vi "Scale Filter before Targeting to FXP.vi"() -> ()   [LabVIEW 2023]
doc: "Demonstrates how to use the DFD Scale Filter VI to scale the coefficients of a filter that has an IIR Cascaded Second-Order Sections Form structure. By scaling the filter coefficients, you can achieve an optimal fixed-point filter design.\n\nComplete the following steps to use this VI.\n1) Specify an IIR Cascaded Second-Order Sections Form structure in the <B>Target Structure</B> input.\n2) Verify that the <B>Scale Filter?</B> value is False.\n3) Run the VI.\n4) Observe the magnitude response, mean squared error (MSE) value, and coefficients report.\n5) Set the <B>Scale Filter?</B> value to True.\n6) Run this VI again. \n7) Observe the MSE value and coefficients report to learn the effect of scaling the filter coefficients before quantizing and modeling a fixed-point filter."
uses:
  <vilib>/addons/Digital Filter Design/_Objects.llb/DFD Quantization Sources.ctl
  <vilib>/addons/Digital Filter Design/_Objects.llb/DFD Coef Norm Type.ctl
  <vilib>/addons/Digital Filter Design/FXPModel.llb/DFD FXP Quantize Coef (Easy).vi
  <vilib>/addons/Digital Filter Design/Analysis.llb/DFD Plot Freq Response (Linear-Spaced).vi
  <vilib>/addons/Digital Filter Design/FXPModel.llb/DFD FXP Get Quantizer (One).vi
  <vilib>/addons/Digital Filter Design/Process.llb/DFD Filtering (Array).vi
  <vilib>/Utility/VariantDataType/GetNumericFxpInfo.vi
  <vilib>/addons/Digital Filter Design/FXPSim.llb/dfd_Check Input FXP Settings.vi
  <vilib>/addons/Digital Filter Design/FXPSim.llb/dfd_Check SRate Simulation Integer Input.vi
  <vilib>/addons/Digital Filter Design/FXPSim.llb/dfd_FXP Simu.vi
  <vilib>/addons/Digital Filter Design/_Objects.llb/DFD FXP Statistics Data.ctl
  <vilib>/addons/Digital Filter Design/FXPSim.llb/SimXnode/DFD FXP Simulation.xnode
  <vilib>/addons/Digital Filter Design/_Objects.llb/DFD Filter Obj.ctl
  <vilib>/addons/Digital Filter Design/_Objects.llb/DFD Filter Coef.ctl
  <vilib>/addons/Digital Filter Design/_Objects.llb/DFD Filter Structure Type Selector.ctl
  <vilib>/addons/Digital Filter Design/_Objects.llb/dfd_Internal Quantization Settings.ctl
  <vilib>/addons/Digital Filter Design/_Objects.llb/dfd_Internal Quantization Srcs.ctl
  <vilib>/addons/Digital Filter Design/NI_DigFilterLicensed.lvlib
  <vilib>/Analysis/NI_AALPro.lvlib
  <vilib>/Analysis/NI_AALBase.lvlib
  <vilib>/addons/Digital Filter Design/NI_DigFilter_FXP.lvlib
  <vilib>/Utility/VariantDataType/VariantType.lvlib
panel:
  out "MSE":dbl format="%.6g"
  out "Coefficients Report":string
  out "Magnitude Response":cluster{"f0":dbl, "df":dbl, "values":dbl[]}[](graph)
  in  "Scale Filter?":bool
  out "Error Message":string
  in  "Target Structure":u16(ring)=12 items=["FIR Direct Form"=1, "FIR Direct Form Transposed"=2, "FIR Symmetric"=3, "FIR Antisymmetric"=4, "IIR Direct Form I"=5, "IIR Direct Form I Transposed"=6, "IIR Direct Form II"=7, "IIR Direct Form II Transposed"=8, "IIR Cascaded Second-Order Sections Form I"=9, "IIR Cascaded Second-Order Sections Form I Transposed"=10, "IIR Cascaded Second-Order Sections Form II"=11, "IIR Cascaded Second-Order Sections Form II Transposed"=12, "Lattice Allpass (basic sections)"=13, "Lattice Allpass (one multiplier sections)"=14, "Lattice Allpass (normalized sections)"=15, "Lattice AR (basic sections)"=16, "Lattice AR (one multiplier sections)"=17, "Lattice AR (normalized sections)"=18, "Lattice MA (minimum phase)"=19, "Lattice MA (maximum phase)"=20, "Lattice ARMA (basic sections)"=21, "Lattice ARMA (one multiplier sections)"=22, "Lattice ARMA (normalized sections)"=23]
  out "Filtering Results":dbl[][](graph)
  # "Select Help>>Show Context Help and move the cursor over the VI icon for more information."
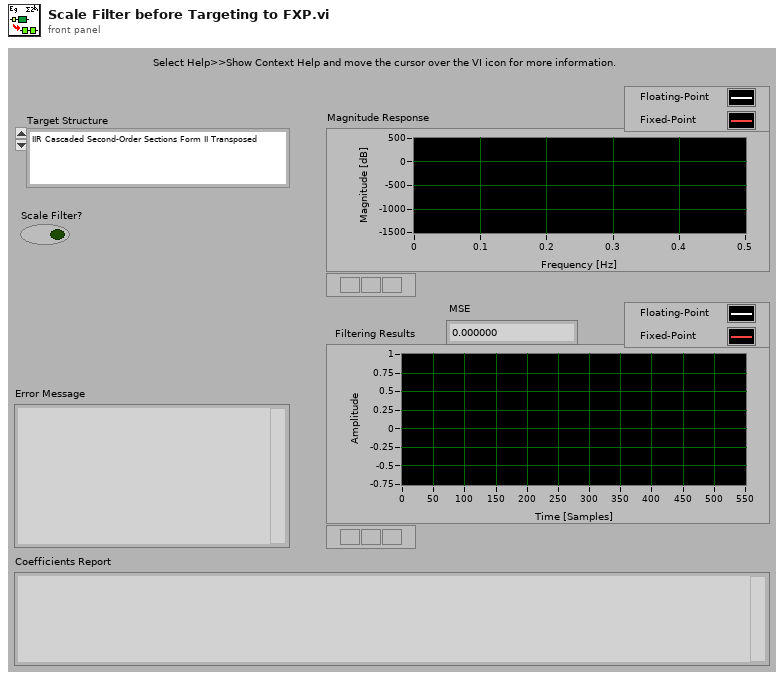
[diagram p1: front panel]
types:
  T1 = typedef "NI_DigFilterLicensed.lvlib/DFD Quantization Sources.ctl" = u16
  T2 = typedef "NI_DigFilterLicensed.lvlib/DFD Filter Obj.ctl" = cluster{"mSRate_Fs":dbl, "mSRate_Version":string, "mSRate_Comments":string, "mSRate_OrgCoef":T3, "mSRate_CurCoef":T3, "mSRate_Quantized?":bool, "mSRate_QCoef":T3, "mSRate_QSettings":T5[], "mSRate_Order":i32, "mSRate_Scaling":cluster{"mSRate_ScaleByPowerOf2?":bool, "mSRate_ScaleType":T7}}
  T3 = typedef "NI_DigFilterLicensed.lvlib/DFD Filter Coef.ctl" = cluster{"type":T4, "gain":dbl, "coef a (k)":dbl[], "coef b (v)":dbl[]}
  T4 = typedef "NI_DigFilterLicensed.lvlib/DFD Filter Structure Type Selector.ctl" = enum16{"Undefined", "FIR Direct Form", "FIR Direct Form Transposed", "FIR Symmetric", "FIR Antisymmetric", "IIR Direct Form I", "IIR Direct Form I Transposed", "IIR Direct Form II", "IIR Direct Form II Transposed", "IIR Cascaded Second Order Sections Form I", "IIR Cascaded Second Order Sections Form I Transposed", "IIR Cascaded Second Order Sections Form II", "IIR Cascaded Second Order Sections Form II Transposed", "Lattice Allpass (basic sections)", "Lattice Allpass (one multiplier sections)", "Lattice Allpass (normalized sections)", "Lattice AR (basic sections)", "Lattice AR (one multiplier sections)", "Lattice AR (normalized sections)", "Lattice MA (minimum phase)", "Lattice MA (maximum phase)", "Lattice ARMA (basic sections)", "Lattice ARMA (one multiplier sections)", "Lattice ARMA (normalized sections)"}
  T5 = typedef "NI_DigFilterLicensed.lvlib/dfd_Internal Quantization Settings.ctl" = cluster{"source":T6, "wl":i16, "iwl":i16, "overflow mode":enum16{"Saturation", "Wrap"}, "rounding mode":enum16{"Nearest", "Truncation"}, "signed?":bool}
  T6 = typedef "NI_DigFilterLicensed.lvlib/dfd_Internal Quantization Srcs.ctl" = u16
  T7 = typedef "NI_DigFilterLicensed.lvlib/DFD Coef Norm Type.ctl" = enum16{"No Norm", "Time Domain 1-Norm", "Time Domain 2-Norm", "Time Domain Inf-Norm"}
  T8 = typedef "NI_DigFilterLicensed.lvlib/DFD Quantization Settings.ctl" = cluster{"source":T1, "wl":i16, "iwl":i16, "overflow mode":enum16{"Saturation", "Wrap"}, "rounding mode":enum16{"Nearest", "Truncation"}, "signed?":bool}
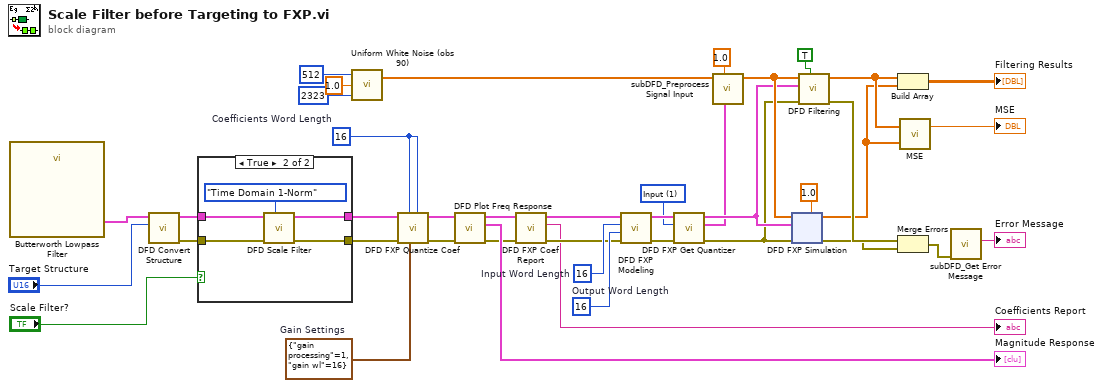
[diagram p0: block diagram]
diagram:
  w3 = T1 1 items=["Coefficients a/k"=0, "Coefficients b/v"=7, "Input"=1, "Output"=2, "Multiplicand"=3, "Product"=4, "Sum"=5, "Delay"=6] ("quantizer source")
  w27 = i16 16  # Output Word Length
  w28 = i16 16  # Input Word Length
  w29 = i16 16  # Coefficients Word Length
  w30 = cluster{"gain processing":u16, "gain wl":i16} {"gain processing"=1, "gain wl"=16}  # Gain Settings
  n1 = call "Butterworth Lowpass Filter"() -> ("filter out"=w1:T2)  [unwired: 1 in, 10 out]
  n2 = call <vilib>:"DFD Convert Structure.vi"("target structure"="Target Structure", "filter in"=w1) -> ("error out"=w34:errorcluster, "filter out"=w35:T2)  [unwired: 1 in, 7 out]
  n3 = case shown="True" "Scale Filter?" {
    tunnel: w35 -> [w43 w47]
    tunnel: w34 -> [w42 w46]
    tunnel: [w43 w45] -> w32
    tunnel: [w42 w44] -> w31
    frame False {
    }
    frame True {
      n4 = call <vilib>:"DFD Scale Filter.vi"("scale type"=DFD_Coef_Norm_Type."Time Domain 1-Norm", "error in (no error)"=w46, "filter in"=w47) -> ("error out"=w44:errorcluster, "filter out"=w45:T2)  [unwired: 7 out]
    }
  }
  n5 = call <vilib>:"Uniform White Noise (obs 90).vi"("seed"=2323, "amplitude"=1.0, "samples"=512) -> ("uniform white noise"=w10:dbl[])  [unwired: 1 out]
  n6 = call-poly <vilib>:"DFD FXP Quantize Coef.vi"("coefficients b/v word length"=w29, "gain settings"=w30, "coefficients a/k word length"=w29, "error in (no error)"=w31, "filter in"=w32) -> ("error out"=w25:errorcluster, "filter out"=w26:T2)  [unwired: 5 out]
  n7 = call-poly <vilib>:"DFD Plot Freq Response.vi"("error in (no error)"=w25, "filter in"=w26) -> ("error out"=w21:errorcluster, "magnitude response"=→"Magnitude Response":cluster{"f0":dbl, "df":dbl, "values":dbl[]}[], "filter out"=w23:T2)  [unwired: 6 in, 1 out]
  n8 = call <vilib>:"DFD FXP Coef Report.vi"("error in (no error)"=w21, "filter in"=w23) -> ("error out"=w20:errorcluster, "coefficients report"=→"Coefficients Report":string, "filter out"=w22:T2)  [unwired: 7 out]
  n9 = call <vilib>:"DFD FXP Modeling.vi"("error in (no error)"=w20, "output word length"=w27, "input word length"=w28, "filter in"=w22) -> ("error out"=w5:errorcluster, "filter out"=w7:T2)  [unwired: 3 in, 3 out]
  n10 = call-poly <vilib>:"DFD FXP Get Quantizer.vi"("error in (no error)"=w5, "quantizer source"=w3, "filter in"=w7) -> ("error out"=w4:errorcluster, "quantizer"=w2:T8, "filter out"=w6:T2)  [unwired: 6 out]
  n11 = call <vilib>:"subDFD_Preprocess Signal Input.vi"("input quantizer"=w2, "input range"=1.0, "x"=w10) -> ("q[x]"=w9:dbl[])  [unwired: 8 out]
  n12 = xnode "DFD FXP Simulation"("input range"=1.0, "error in (no error)"=w4, "filter in"=w6, "signal in"=w9) -> ("error out"=w15:errorcluster, "DBL signal out"=w12:dbl[])  [unwired: 1 in, 3 out]
  n13 = call-poly <vilib>:"DFD Filtering.vi"("init? (F)"=TRUE, "error in (no error)"=w4, "filter"=w6, "signal in"=w9) -> ("error out"=w16:errorcluster, "signal out"=w13:dbl[])  [unwired: 6 out]
  n14 = Build Array(w13, w12) -> (→"Filtering Results":dbl[][])
  n15 = Merge Errors(w16, w15) -> (w14:errorcluster)
  n16 = call <vilib>:"MSE.vi"("X Values"=w12, "Y Values"=w13) -> ("mse"=→"MSE":dbl)  [unwired: 1 out]
  n17 = call <vilib>:"subDFD_Get Error Message.vi"("error in (no error)"=w14) -> ("Error Message"=→"Error Message":string)  [unwired: 10 out]
